vi "Toggle.vi"() -> (3 "Boolean":bool)   [LabVIEW 2014]
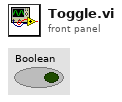
[diagram p1: front panel]
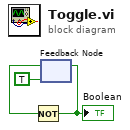
[diagram p0: block diagram]
diagram:
  n1 = feedback #1(TRUE) -> (w2:bool)
  n2 = Not(x=w2) -> (.not. x?=w3:bool)
  "Boolean" <- w3
  n3 = feedback-in #1(w3) -> ()
